vi "Configure GPIB Controller.vi"(8 "error in (no error)":errorcluster, 9 "Read-after-Write?":bool, 10 "Address":u32=1, 11 "VISA Refnum in":refnum<visa-resource-name>) -> (0 "error out":errorcluster, 3 "VISA Refnum out":refnum<visa-resource-name>)   [LabVIEW 2015]
doc: "Sets the Prologix GPIB-USB Controller read-after-write function and the address to the input values."
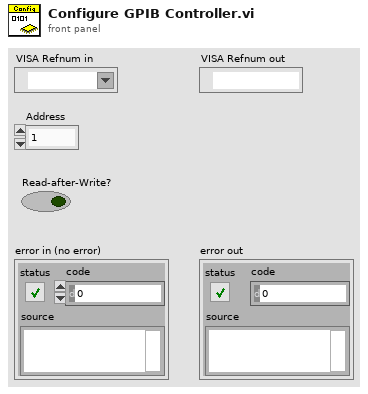
[diagram p1: front panel]
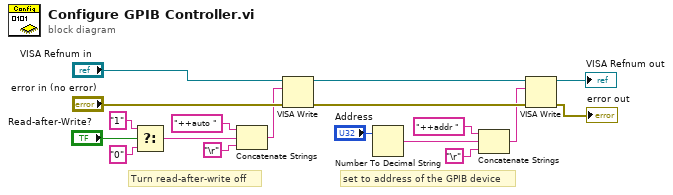
[diagram p0: block diagram]
diagram:
  # "Turn read-after-write off"
  # "set to address of the GPIB device"
  n1 = Select(t="1", s="Read-after-Write?", f="0") -> (s? t:f=w2:string)
  n2 = Concatenate Strings("++auto " ("write buffer"), w2, "\r") -> (w14:string)
  n3 = VISA Write(VISA resource name="VISA Refnum in", write buffer=w14, error in (no error)="error in (no error)") -> (VISA resource name out=w17:refnum<visa-resource-name>, error out=w18:errorcluster)  [unwired: 1 out]
  n4 = Number To Decimal String(number="Address") -> (decimal integer string=w12:string)  [unwired: 1 in]
  n5 = Concatenate Strings("++addr " ("write buffer"), w12, "\r") -> (w6:string)
  n6 = VISA Write(VISA resource name=w17, write buffer=w6, error in (no error)=w18) -> (VISA resource name out=→"VISA Refnum out":refnum<visa-resource-name>, error out=→"error out":errorcluster)  [unwired: 1 out]
